vi "IndustrialWriteCustomRule.vi"(11 "IsImmediate":bool) -> (3 "New Custom Rule":string)   [LabVIEW 2017, in "NI_Variable.lvlib"]
uses:
  <vilib>/variable/NI_Variable.lvlib
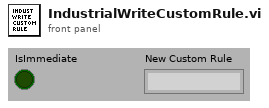
[diagram p1: front panel]
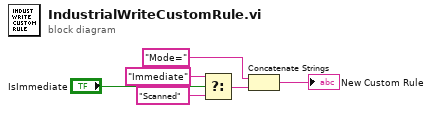
[diagram p0: block diagram]
diagram:
  n1 = Select(t="Immediate", s="IsImmediate", f="Scanned") -> (s? t:f=w3:string)
  n2 = Concatenate Strings("Mode=" ("regular expression"), w3) -> (→"New Custom Rule":string)
